vi "GetStructuringElement.vi"(8 "error in":errorcluster, 9 "Anchor":T2={"X"=-1, "Y"=-1}, 10 "Size":T2={"X"=5, "Y"=5}, 11 "MorphShapes":T1) -> (0 "error out":errorcluster, 3 "structuringElement":u8[][](array[numeric]))   [LabVIEW 2020, in "OpenLvVision_OpenCv.lvlib"]
doc: "Returns a structuring element of the specified size and shape for morphological operations."
uses:
  OpenLvVision_OpenCv.lvlib
  TypeDef/Point/2D_PointI32.ctl
  TypeDef/MorphShapes.ctl
  Dlls/OlvOpenCvWrapper.dll
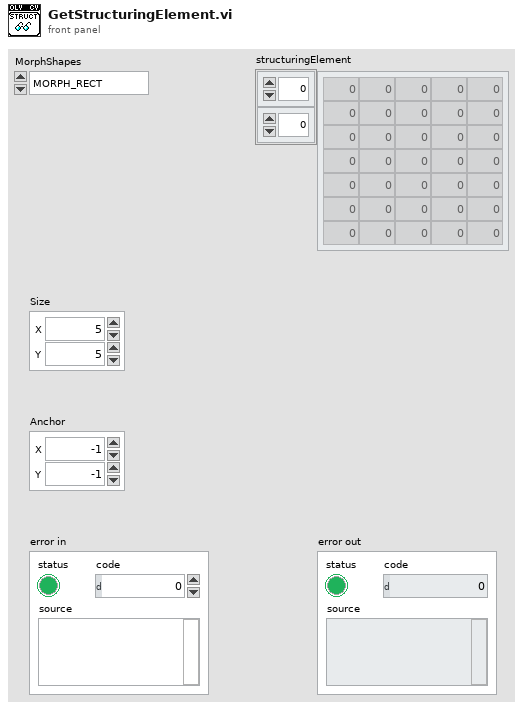
[diagram p1: front panel]
types:
  T1 = typedef "OpenLvVision_OpenCv.lvlib/MorphShapes.ctl" = enum16{"MORPH_RECT", "MORPH_CROSS", "MORPH_ELLIPSE"}
  T2 = typedef "OpenLvVision_OpenCv.lvlib/2D_PointI32.ctl" = cluster{"X":i32, "Y":i32}
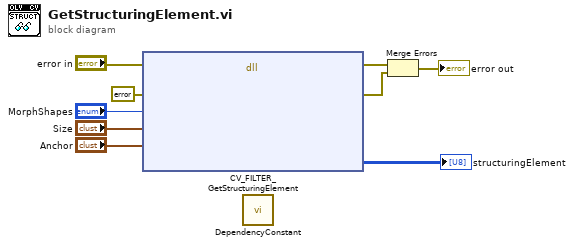
[diagram p0: block diagram]
diagram:
  n1 = dll-call lib="C:/Users/lukas/Downloads/OpenLvVision_OpenCv/SourceCode/LabView/OpenLvVision_OpenCv/Dlls/OlvOpenCvWrapper.dll" fn="CV_FILTER_GetStructuringElement"(error in="error in", "Error"=errorcluster {"status"=FALSE, "code"=0, "source"=""} ("error constant"), "shape"="MorphShapes", "kSize"="Size", "anchor"="Anchor") -> (error out=w8:errorcluster, "Error"=w5:errorcluster, "structuringElement"=→"structuringElement":u8[][])  [unwired: 7 in, 1 out]
  n2 = call "DependencyConstant.vi"() -> ()  [unwired: 12 in]
  n3 = Merge Errors(w8, w5) -> (→"error out":errorcluster)
